vi "Determine_if_transformation is possible.vi"(6 "NUmber of Sessions Prior to Current":i32, 9 "Session_list":T2(array[cluster]), 10 "numberFidsCurrentSession":i32, 11 "CollectionOfPoints":T1[](array[typedef])) -> (2 "Fiducial count":u32[](array[numeric]), 3 "AtLeast3MatchingFids":bool)   [LabVIEW 2011]
uses:
  cm2nm_coordinate_information_v2.ctl
  cm2nm_sample_set.ctl
  Instrument_type_enum_v2.ctl
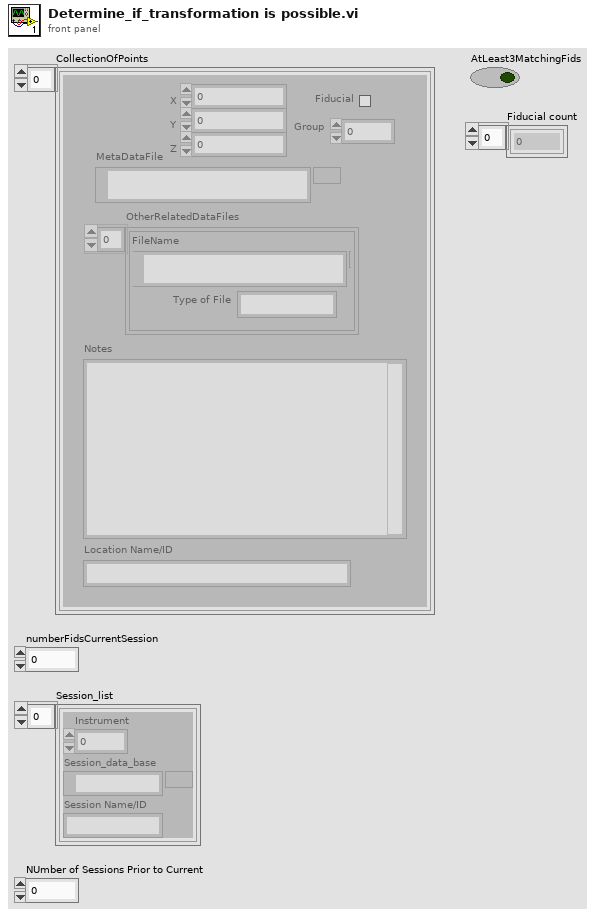
[diagram p1: front panel]
types:
  T1 = typedef "cm2nm_coordinate_information_v2.ctl" = cluster{"MetaDataFile":path, "X":dbl, "Y":dbl, "Z":dbl, "Group":i32, "Rotation":dbl[unit], "Fiducial":bool, "Magnification":dbl, "Working_Distance":dbl, "Notes":string, "Location Name/ID":string, "OtherRelatedDataFiles":cluster{"Type of File":string, "FileName":path}[], "Available":bool}
  T2 = cluster{"Instrument":u16, "Session_data_base":path, "Session Name/ID":string}[]
  T3 = typedef "cm2nm_sample_set.ctl" = cluster{"CollectionOfPoints":T1[], "Instrument":T4, "CollectionFile":path, "Session Name/ID":string, "SessionNotes":string}
  T4 = typedef "Instrument_type_enum_v2.ctl" = enum16{"Unknown", "Philips FEI SEM IRC", "JEOL 7000F EML_MFC", "MXRD MFC", "JEOL_EPMA"}
  T5 = cluster{"Instrument":u16, "Session_data_base":path, "Session Name/ID":string}
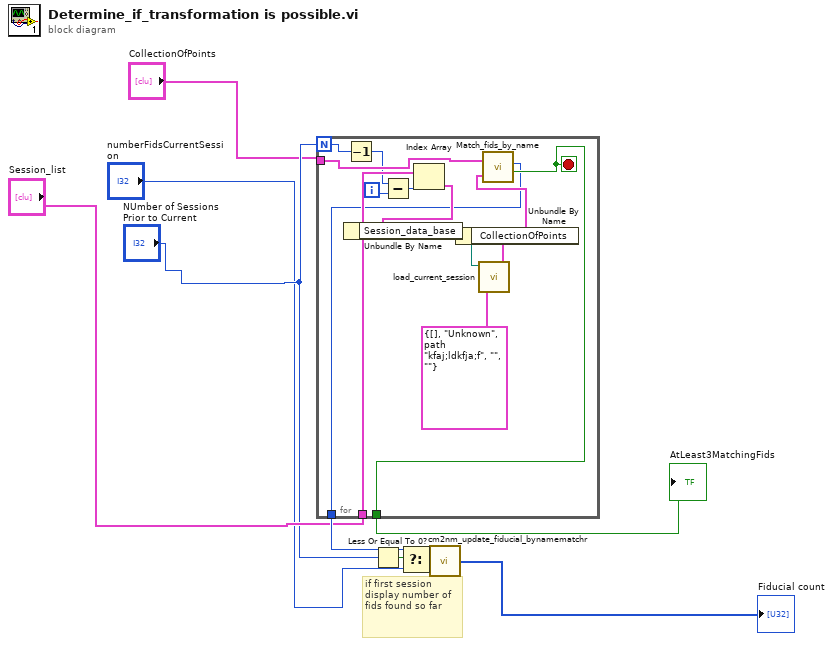
[diagram p0: block diagram]
diagram:
  # "if first session\ndisplay number of\nfids found so far"
  n1 = for {
    N: "NUmber of Sessions Prior to Current" -> [w20]
    tunnel: "Session_list" -> [w21]
    tunnel: "CollectionOfPoints" -> [w22]
    tunnel: [w11] -> w5
    tunnel: [w10] -> w8
    i -> [w18]
    stop <- w11 stop-if-true
    n2 = Decrement(x=w20) -> (x-1=w19:i32)
    n3 = Subtract(x=w19, y=w18) -> (x-y=w17:i32)
    n4 = Index Array(array=w21, index=w17) -> (element=w16:T5)
    n5 = Unbundle By Name(w16) -> ("Session_data_base"=w15:path)
    n6 = call "load_current_session.vi"("Current Session Information"=T3 {"CollectionOfPoints"=[], "Instrument"=enum."Unknown", "CollectionFile"=path "kfaj;ldkfja;f", "Session Name/ID"="", "SessionNotes"=""}, "just a file"=w15) -> ("Sample Set"=w13:T3)  [unwired: 2 in, 2 out]
    n7 = Unbundle By Name(w13) -> ("CollectionOfPoints"=w12:T1[])
    n8 = call "Match_fids_by_name.vi"("CurrentSessionDataSet"=w22, "ReferenceSessionDataSet"=w12) -> ("NumberOfNameMatch"=w10:i32, "AtLeast3"=w11:bool)  [unwired: 2 out]
  }
  "AtLeast3MatchingFids" <- w5
  n9 = Less Or Equal To 0?(x="NUmber of Sessions Prior to Current") -> (x <= 0?=w7:bool)
  n10 = Select(t=w8, s=w7, f="numberFidsCurrentSession") -> (s? t:f=w9:i32)
  n11 = call "cm2nm_update_fiducial_bynamematchr.vi"("numbermatchedbyname"=w9) -> ("Array"=→"Fiducial count":u32[])
